vi "Get Zernike Coefficients.vi"(8 "error in (no error)":errorcluster, 11 "HasoSlopes in":refnum<class "HasoSlopes.lvclass">) -> (0 "error out":errorcluster, 2 "Coefficients":sgl[](array[numeric]), 3 "HasoSlopes out":refnum<class "HasoSlopes.lvclass">)   [LabVIEW 2020]
uses:
  WaveKit/Classes/HasoSlopes/HasoSlopes.lvclass
  WaveKit/Classes/Pupil/Pupil.lvclass
  WaveKit/Classes/ModalCoef/ModalCoef.lvclass
panel:
  out "Zernicke Pupil":i32[][](graph)
  in  "ModalCoef in":refnum<class "ModalCoef.lvclass">
  in  "Pupil in":refnum<class "Pupil.lvclass">
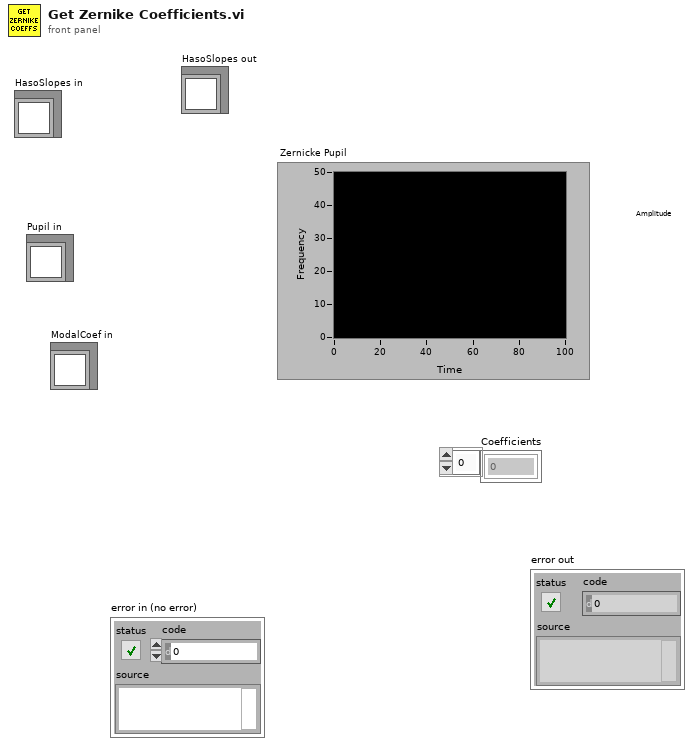
[diagram p1: front panel]
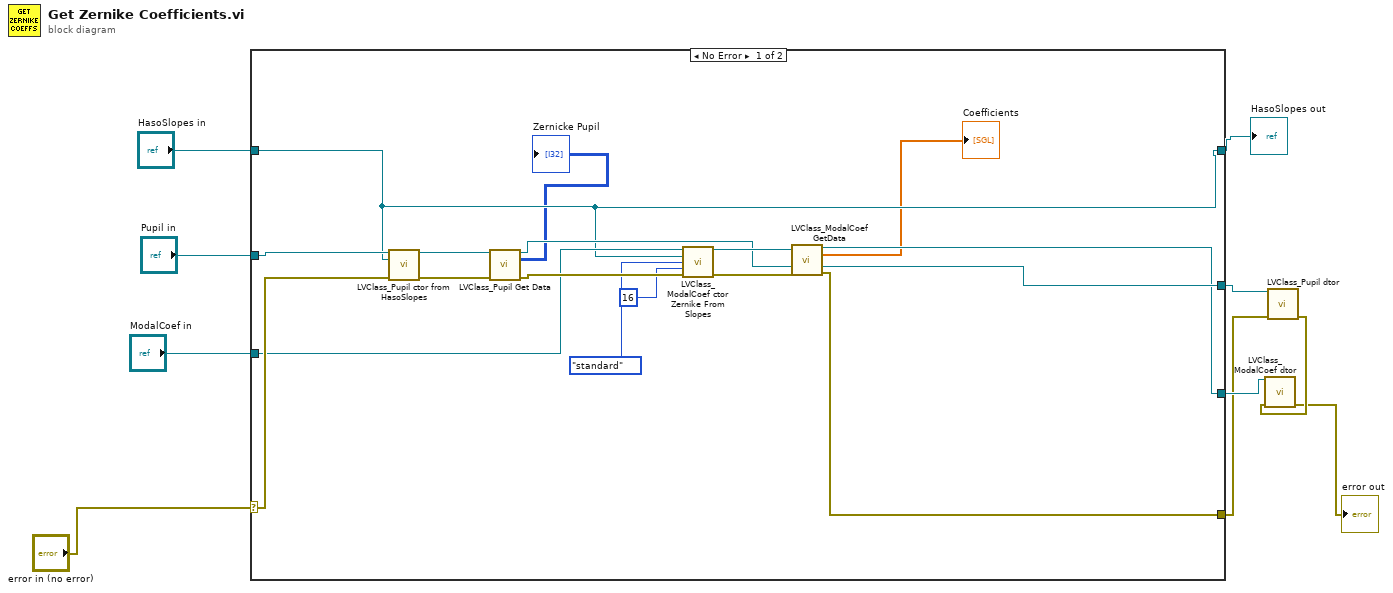
[diagram p0: block diagram]
diagram:
  n1 = case shown="No Error" "error in (no error)" {
    selector: "error in (no error)" -> [w25 w28]
    tunnel: "HasoSlopes in" -> [w16 w31]
    tunnel: "Pupil in" -> [w27 w30]
    tunnel: "ModalCoef in" -> [w22 w29]
    tunnel: [w16 w31] -> w6
    tunnel: [w14 w30] -> w4
    tunnel: [w13 w29] -> w5
    tunnel: [w15 w28] -> w3
    frame No Error {
      n2 = call "LVClass_Pupil ctor from HasoSlopes.vi"("Pupil (const)"=w27, "HasoSlopes"=w16, "error in (no error)"=w25) -> ("Pupil (new)"=w26:refnum<class "Pupil.lvclass">, "error out"=w24:errorcluster)  [unwired: 10 in, 1 out]
      n3 = call "LVClass_Pupil Get Data.vi"("Pupil in"=w26, "error in (no error)"=w24) -> ("Pupil out"=w17:refnum<class "Pupil.lvclass">, "Data"=→"Zernicke Pupil":i32[][], "error out"=w23:errorcluster)  [unwired: 11 in]
      n4 = call "LVClass_ModalCoef ctor Zernike From Slopes.vi"("ModalCoef (const)"=w22, "HasoSlopes"=w16, "normalization"=enum16{"standard", "rms"}."standard", "nb_coefs"=u32 16, "error in (no error)"=w23) -> ("ModalCoef (new)"=w19:refnum<class "ModalCoef.lvclass">, "error out"=w18:errorcluster)  [unwired: 9 in]
      n5 = call "LVClass_ModalCoef GetData.vi"("ModalCoef in"=w19, "Pupil.lvclass"=w17, "error in (no error)"=w18) -> ("ModalCoef out"=w13:refnum<class "ModalCoef.lvclass">, "coef"=→"Coefficients":sgl[], "Pupil.lvclass (dup)"=w14:refnum<class "Pupil.lvclass">, "error out"=w15:errorcluster)  [unwired: 8 in, 1 out]
    }
    frame Error {
    }
  }
  "HasoSlopes out" <- w6
  n6 = call "LVClass_Pupil dtor.vi"("Pupil in"=w4, "error in (no error)"=w3) -> ("error out"=w2:errorcluster)  [unwired: 12 in, 1 out]
  n7 = call "LVClass_ModalCoef dtor.vi"("ModalCoef in"=w5, "error in (no error)"=w2) -> ("error out"=→"error out":errorcluster)  [unwired: 12 in, 1 out]
